vi "gjson_Parse.vi"(8 "error in":errorcluster, 10 "JSON String In":string, 11 "JSON Cluster":variant) -> (0 "error out":errorcluster, 3 "JSON Cluster Out":variant)   [LabVIEW 2015, in "Json2Labv.lvlib"]
uses:
  Json2Labv.lvlib
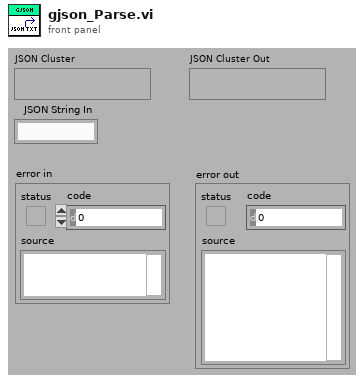
[diagram p1: front panel]
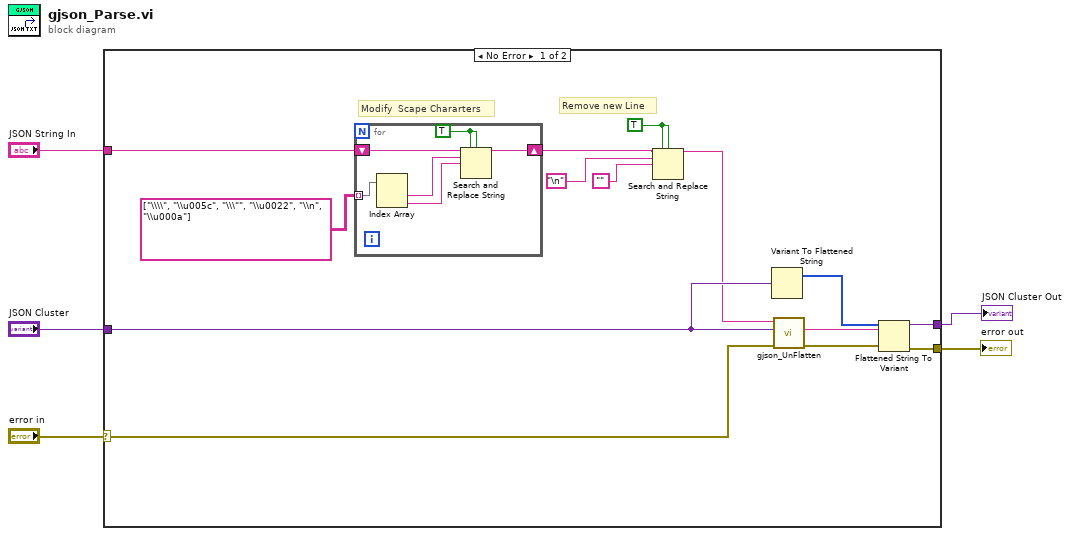
[diagram p0: block diagram]
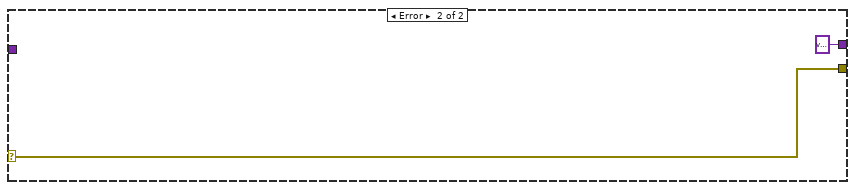
[diagram p2: hidden frame]
diagram:
  n1 = case shown="No Error" "error in" {
    selector: "error in" -> [w6 w27]
    tunnel: "JSON Cluster" -> [w14 _]
    tunnel: [w12 w27] -> w4
    tunnel: [w11 variant ("Variant")] -> w3
    tunnel: "JSON String In" -> [w10 _]
    frame No Error {
      w8 = TRUE ("replace all? (F)")
      # "Remove new Line"
      # "Modify  Scape Chararters"
      n2 = for {
        shift-right: [w24] -> w9
        shift-left: w10 -> [w25]
        tunnel: string[][] [["\\\\", "\\u005c"], ["\\\"", "\\u0022"], ["\\n", "\\u000a"]] -> [w23] mode=indexing
        w20 = TRUE ("replace all? (F)")
        n3 = Index Array(array=w23) -> (element #1=w22:string, element #2=w21:string)  [unwired: 2 in]
        n4 = Search and Replace String(replace all?=w20, case sensitive?=w20, input string=w25, search string=w22, replace string=w21) -> (result string=w24:string)  [unwired: 3 in, 3 out]
      }
      n5 = Search and Replace String(replace all?=w8, case sensitive?=w8, input string=w9, search string="\n", replace string="") -> (result string=w7:string)  [unwired: 3 in, 3 out]
      n6 = Variant To Flattened String(Variant=w14) -> (1:w13:i16[])  [unwired: 1 out]
      n7 = call "gjson_UnFlatten.vi"("error in"=w6, "Variant"=w14, "JSON String In"=w7) -> ("error out"=w16:errorcluster, "UnFlattenData Out"=w15:string)  [unwired: 6 in, 1 out]
      n8 = Flattened String To Variant(4:w16, 6:w15, 7:w13) -> (0:w12:errorcluster, 3:w11:variant)
    }
    frame Error {
    }
  }
  "error out" <- w4
  "JSON Cluster Out" <- w3
